vi "datatojson.vi"() -> (3 "json":string[](array[string]))   [LabVIEW 2016, in "工况数据上传.lvlib"]
panel:
  out "data":T1={"time"="2021-05-08 14-02-02", "data"={"ups"={"ups"={"input_voltage"=0.0, "input_frequency"=0.0, "output_voltage"=0.0, "output_current"=0.0, "output_frequency"=0.0, "output_active_power"=0.0, "output_apparent_power"=0.0, "load_rate"=0.0, "cabinet_temperature"=0.0, "battery_voltage"=0.0, "remaining_battery_capacity"=0.0, "power_on_status"="", "power_supply_mode"="", "fault"=FALSE, "battery_low_voltage"=FALSE, "mains_supply_abnormality"=FALSE}, "启用"=FALSE}, "air_conditioner"={"air_conditioner"={"cabinet_temperature"=0.0, "air_supply_temperature"=0.0, "voltage"=0.0, "current"=0.0, "compressor_status"="", "Internal_fan_status"="", "external_fan_status"="", "heating_state"="", "refrigeration_state"=FALSE, "high_temperature_alarm"=FALSE, "low_temperature_alarm"=FALSE, "heater_fault"=FALSE, "temperature_sensor_fault"=FALSE, "high_voltage_alarm"=FALSE, "low_voltage_alarm"=FALSE, "refrigeration_start_point"=0.0, "refrigeration_sensitive_point"=0.0, "heating_start_point"=0.0, "heating_sensitive_point"=0.0, "high_temperature_alarm_point"=0.0, "low_temperature_alarm_point"=0.0}, "启用"=FALSE}, "smoke_sensor"={"smoke_sensor"={"trigger_alarm"=FALSE}, "启用"=FALSE}, "water_immersion_sensor"={"water_immersion_sensor"={"trigger_alarm"=FALSE}, "启用"=FALSE}, "temperature_and_humidity_sensor"={"temperature_and_humidity_sensor"={"current_temperature"=0.0, "current_humidity"=0.0, "room_temperature_alarm"=FALSE, "humidity_alarm"=FALSE}, "启用"=FALSE}, "gps"={"gps"={"current_longitude"=0.0, "current_latitude"=0.0, "launch_longitude"=0.0, "launch_latitude"=0.0, "shift_alarm"=FALSE}, "启用"=FALSE}, "solar_controller"={"solar_controller"={"array_voltage"=0.0, "array_current"=0.0, "generating_power"=0.0, "battery_voltage"=0.0, "battery_current"=0.0, "ceiling_voltage"=0.0, "minimum_voltage"=0.0, "battery_temperature"=0.0, "remaining_battery_capacity"=0.0, "load_voltage"=0.0, "load_current"=0.0, "load_power"=0.0, "equipment_temperature"=0.0, "accumulated_electricity_consumption_of_the_day"=0.0, "accumulated_electricity_consumption_of_the_current_month"=0.0, "accumulated_electricity_consumption_in_the_current_year"=0.0, "total_accumulated_power_consumption"=0.0, "accumulated_charging_capacity_of_the_day"=0.0, "accumulated_charging_amount_of_the_current_month"=0.0, "accumulated_charging_capacity_of_the_current_year"=0.0, "total_cumulative_charge"=0.0}, "启用"=FALSE}, "solar_controller_2"={"solar_controller_2"={"array_voltage"=0.0, "array_current"=0.0, "generating_power"=0.0, "battery_voltage"=0.0, "battery_current"=0.0, "ceiling_voltage"=0.0, "minimum_voltage"=0.0, "battery_temperature"=0.0, "remaining_battery_capacity"=0.0, "load_voltage"=0.0, "load_current"=0.0, "load_power"=0.0, "equipment_temperature"=0.0, "accumulated_electricity_consumption_of_the_day"=0.0, "accumulated_electricity_consumption_of_the_current_month"=0.0, "accumulated_electricity_consumption_in_the_current_year"=0.0, "total_accumulated_power_consumption"=0.0, "accumulated_charging_capacity_of_the_day"=0.0, "accumulated_charging_amount_of_the_current_month"=0.0, "accumulated_charging_capacity_of_the_current_year"=0.0, "total_cumulative_charge"=0.0}, "启用"=FALSE}}} {"data"."air_conditioner"."air_conditioner"."current" format="%#.2g"}
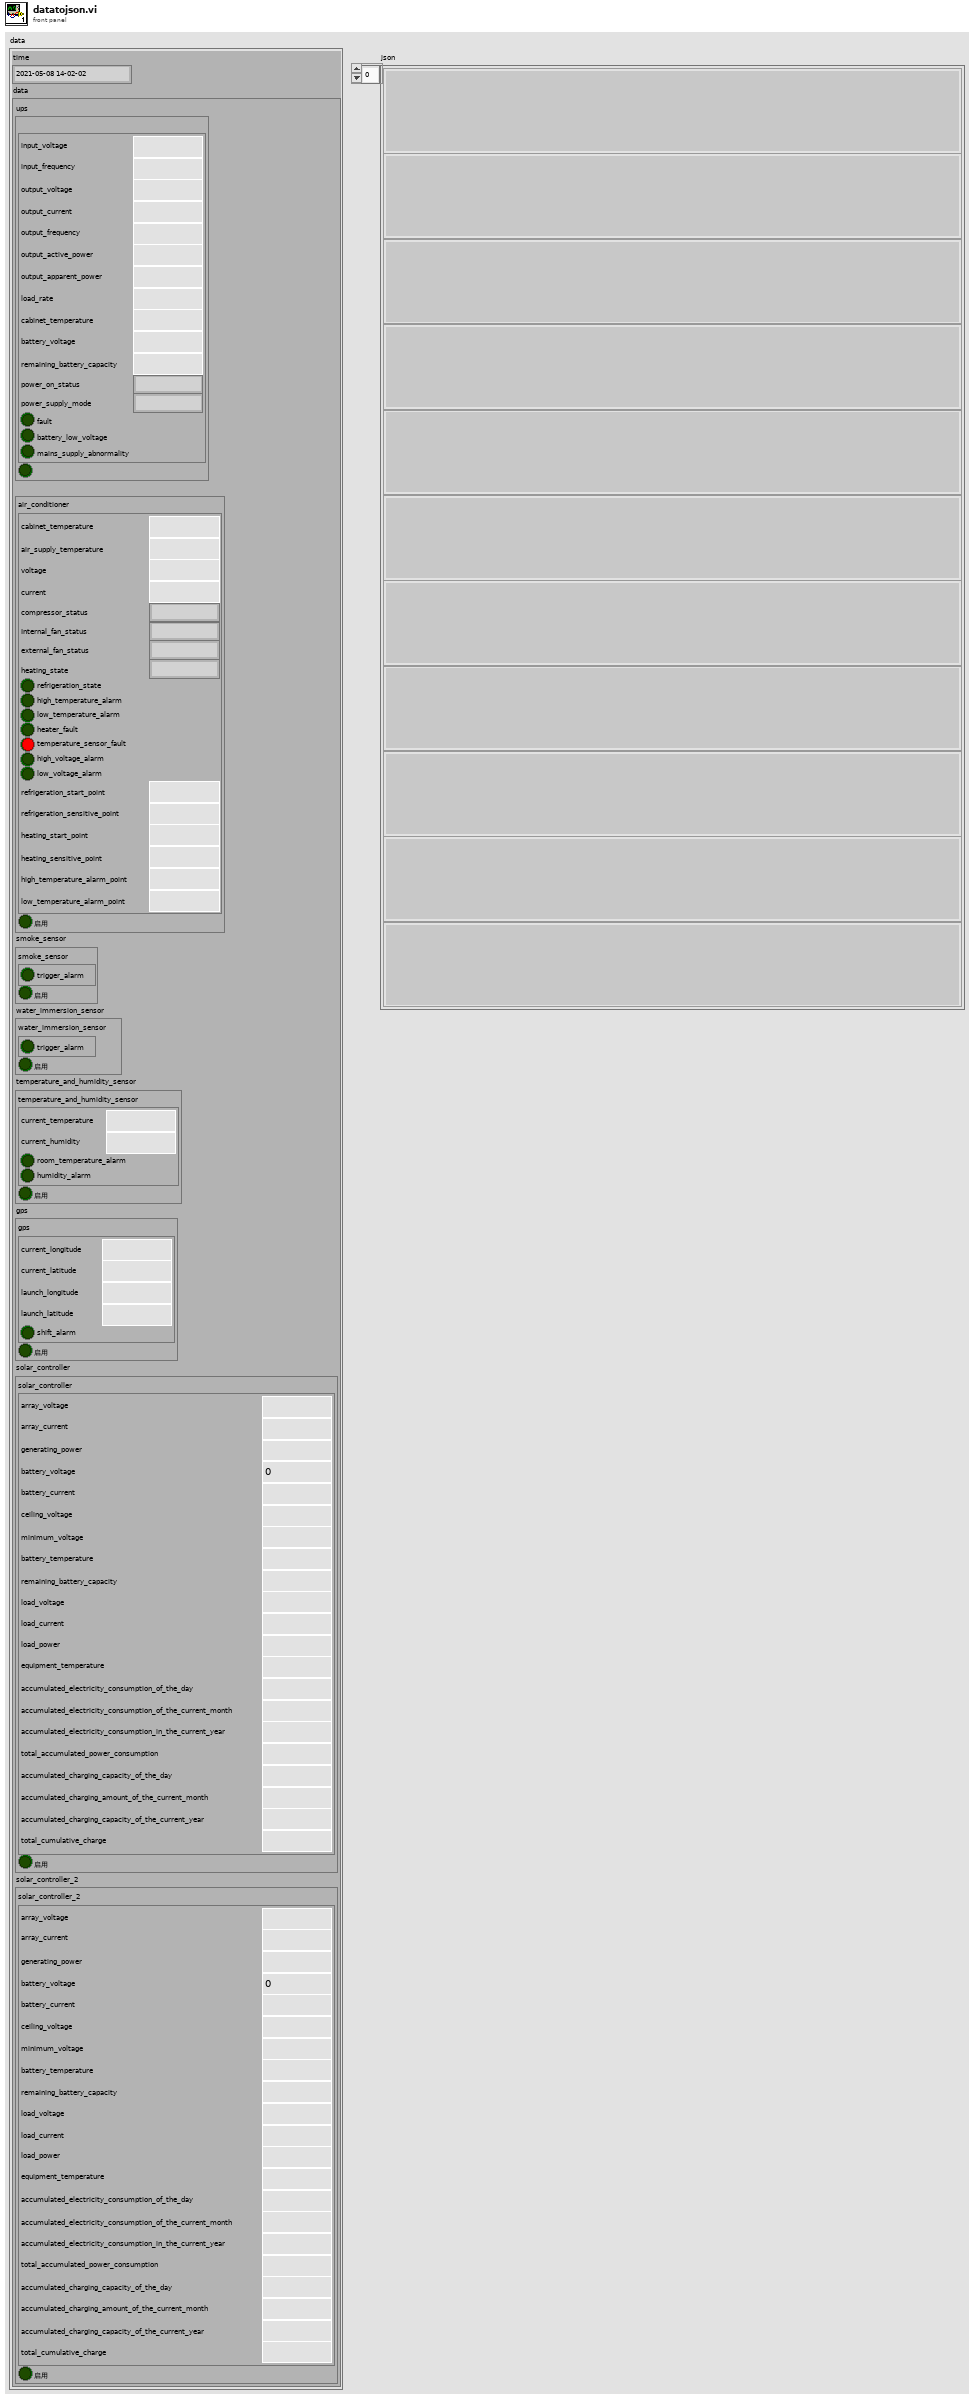
[diagram p1: front panel]
types:
  T1 = typedef "工况数据.ctl" = cluster{"time":string, "data":cluster{"ups":cluster{"ups":cluster{"input_voltage":ext, "input_frequency":ext, "output_voltage":ext, "output_current":ext, "output_frequency":ext, "output_active_power":ext, "output_apparent_power":ext, "load_rate":ext, "cabinet_temperature":ext, "battery_voltage":ext, "remaining_battery_capacity":ext, "power_on_status":string, "power_supply_mode":string, "fault":bool, "battery_low_voltage":bool, "mains_supply_abnormality":bool}, "启用":bool}, "air_conditioner":cluster{"air_conditioner":cluster{"cabinet_temperature":ext, "air_supply_temperature":ext, "voltage":ext, "current":ext, "compressor_status":string, "Internal_fan_status":string, "external_fan_status":string, "heating_state":string, "refrigeration_state":bool, "high_temperature_alarm":bool, "low_temperature_alarm":bool, "heater_fault":bool, "temperature_sensor_fault":bool, "high_voltage_alarm":bool, "low_voltage_alarm":bool, "refrigeration_start_point":ext, "refrigeration_sensitive_point":ext, "heating_start_point":ext, "heating_sensitive_point":ext, "high_temperature_alarm_point":ext, "low_temperature_alarm_point":ext}, "启用":bool}, "smoke_sensor":cluster{"smoke_sensor":cluster{"trigger_alarm":bool}, "启用":bool}, "water_immersion_sensor":cluster{"water_immersion_sensor":cluster{"trigger_alarm":bool}, "启用":bool}, "temperature_and_humidity_sensor":cluster{"temperature_and_humidity_sensor":cluster{"current_temperature":ext, "current_humidity":ext, "room_temperature_alarm":bool, "humidity_alarm":bool}, "启用":bool}, "gps":cluster{"gps":cluster{"current_longitude":ext, "current_latitude":ext, "launch_longitude":ext, "launch_latitude":ext, "shift_alarm":bool}, "启用":bool}, "solar_controller":cluster{"solar_controller":cluster{"array_voltage":ext, "array_current":ext, "generating_power":ext, "battery_voltage":dbl, "battery_current":ext, "ceiling_voltage":ext, "minimum_voltage":ext, "battery_temperature":ext, "remaining_battery_capacity":ext, "load_voltage":ext, "load_current":ext, "load_power":ext, "equipment_temperature":ext, "accumulated_electricity_consumption_of_the_day":ext, "accumulated_electricity_consumption_of_the_current_month":ext, "accumulated_electricity_consumption_in_the_current_year":ext, "total_accumulated_power_consumption":ext, "accumulated_charging_capacity_of_the_day":ext, "accumulated_charging_amount_of_the_current_month":ext, "accumulated_charging_capacity_of_the_current_year":ext, "total_cumulative_charge":ext}, "启用":bool}, "solar_controller_2":cluster{"solar_controller_2":cluster{"array_voltage":ext, "array_current":ext, "generating_power":ext, "battery_voltage":dbl, "battery_current":ext, "ceiling_voltage":ext, "minimum_voltage":ext, "battery_temperature":ext, "remaining_battery_capacity":ext, "load_voltage":ext, "load_current":ext, "load_power":ext, "equipment_temperature":ext, "accumulated_electricity_consumption_of_the_day":ext, "accumulated_electricity_consumption_of_the_current_month":ext, "accumulated_electricity_consumption_in_the_current_year":ext, "total_accumulated_power_consumption":ext, "accumulated_charging_capacity_of_the_day":ext, "accumulated_charging_amount_of_the_current_month":ext, "accumulated_charging_capacity_of_the_current_year":ext, "total_cumulative_charge":ext}, "启用":bool}}}
  T2 = cluster{"ups":cluster{"ups":cluster{"input_voltage":ext, "input_frequency":ext, "output_voltage":ext, "output_current":ext, "output_frequency":ext, "output_active_power":ext, "output_apparent_power":ext, "load_rate":ext, "cabinet_temperature":ext, "battery_voltage":ext, "remaining_battery_capacity":ext, "power_on_status":string, "power_supply_mode":string, "fault":bool, "battery_low_voltage":bool, "mains_supply_abnormality":bool}, "启用":bool}, "air_conditioner":cluster{"air_conditioner":cluster{"cabinet_temperature":ext, "air_supply_temperature":ext, "voltage":ext, "current":ext, "compressor_status":string, "Internal_fan_status":string, "external_fan_status":string, "heating_state":string, "refrigeration_state":bool, "high_temperature_alarm":bool, "low_temperature_alarm":bool, "heater_fault":bool, "temperature_sensor_fault":bool, "high_voltage_alarm":bool, "low_voltage_alarm":bool, "refrigeration_start_point":ext, "refrigeration_sensitive_point":ext, "heating_start_point":ext, "heating_sensitive_point":ext, "high_temperature_alarm_point":ext, "low_temperature_alarm_point":ext}, "启用":bool}, "smoke_sensor":cluster{"smoke_sensor":cluster{"trigger_alarm":bool}, "启用":bool}, "water_immersion_sensor":cluster{"water_immersion_sensor":cluster{"trigger_alarm":bool}, "启用":bool}, "temperature_and_humidity_sensor":cluster{"temperature_and_humidity_sensor":cluster{"current_temperature":ext, "current_humidity":ext, "room_temperature_alarm":bool, "humidity_alarm":bool}, "启用":bool}, "gps":cluster{"gps":cluster{"current_longitude":ext, "current_latitude":ext, "launch_longitude":ext, "launch_latitude":ext, "shift_alarm":bool}, "启用":bool}, "solar_controller":cluster{"solar_controller":cluster{"array_voltage":ext, "array_current":ext, "generating_power":ext, "battery_voltage":dbl, "battery_current":ext, "ceiling_voltage":ext, "minimum_voltage":ext, "battery_temperature":ext, "remaining_battery_capacity":ext, "load_voltage":ext, "load_current":ext, "load_power":ext, "equipment_temperature":ext, "accumulated_electricity_consumption_of_the_day":ext, "accumulated_electricity_consumption_of_the_current_month":ext, "accumulated_electricity_consumption_in_the_current_year":ext, "total_accumulated_power_consumption":ext, "accumulated_charging_capacity_of_the_day":ext, "accumulated_charging_amount_of_the_current_month":ext, "accumulated_charging_capacity_of_the_current_year":ext, "total_cumulative_charge":ext}, "启用":bool}, "solar_controller_2":cluster{"solar_controller_2":cluster{"array_voltage":ext, "array_current":ext, "generating_power":ext, "battery_voltage":dbl, "battery_current":ext, "ceiling_voltage":ext, "minimum_voltage":ext, "battery_temperature":ext, "remaining_battery_capacity":ext, "load_voltage":ext, "load_current":ext, "load_power":ext, "equipment_temperature":ext, "accumulated_electricity_consumption_of_the_day":ext, "accumulated_electricity_consumption_of_the_current_month":ext, "accumulated_electricity_consumption_in_the_current_year":ext, "total_accumulated_power_consumption":ext, "accumulated_charging_capacity_of_the_day":ext, "accumulated_charging_amount_of_the_current_month":ext, "accumulated_charging_capacity_of_the_current_year":ext, "total_cumulative_charge":ext}, "启用":bool}}
  T3 = cluster{"ups":cluster{"input_voltage":ext, "input_frequency":ext, "output_voltage":ext, "output_current":ext, "output_frequency":ext, "output_active_power":ext, "output_apparent_power":ext, "load_rate":ext, "cabinet_temperature":ext, "battery_voltage":ext, "remaining_battery_capacity":ext, "power_on_status":string, "power_supply_mode":string, "fault":bool, "battery_low_voltage":bool, "mains_supply_abnormality":bool}, "启用":bool}
  T4 = cluster{"air_conditioner":cluster{"cabinet_temperature":ext, "air_supply_temperature":ext, "voltage":ext, "current":ext, "compressor_status":string, "Internal_fan_status":string, "external_fan_status":string, "heating_state":string, "refrigeration_state":bool, "high_temperature_alarm":bool, "low_temperature_alarm":bool, "heater_fault":bool, "temperature_sensor_fault":bool, "high_voltage_alarm":bool, "low_voltage_alarm":bool, "refrigeration_start_point":ext, "refrigeration_sensitive_point":ext, "heating_start_point":ext, "heating_sensitive_point":ext, "high_temperature_alarm_point":ext, "low_temperature_alarm_point":ext}, "启用":bool}
  T5 = cluster{"smoke_sensor":cluster{"trigger_alarm":bool}, "启用":bool}
  T6 = cluster{"water_immersion_sensor":cluster{"trigger_alarm":bool}, "启用":bool}
  T7 = cluster{"temperature_and_humidity_sensor":cluster{"current_temperature":ext, "current_humidity":ext, "room_temperature_alarm":bool, "humidity_alarm":bool}, "启用":bool}
  T8 = cluster{"gps":cluster{"current_longitude":ext, "current_latitude":ext, "launch_longitude":ext, "launch_latitude":ext, "shift_alarm":bool}, "启用":bool}
  T9 = cluster{"solar_controller":cluster{"array_voltage":ext, "array_current":ext, "generating_power":ext, "battery_voltage":dbl, "battery_current":ext, "ceiling_voltage":ext, "minimum_voltage":ext, "battery_temperature":ext, "remaining_battery_capacity":ext, "load_voltage":ext, "load_current":ext, "load_power":ext, "equipment_temperature":ext, "accumulated_electricity_consumption_of_the_day":ext, "accumulated_electricity_consumption_of_the_current_month":ext, "accumulated_electricity_consumption_in_the_current_year":ext, "total_accumulated_power_consumption":ext, "accumulated_charging_capacity_of_the_day":ext, "accumulated_charging_amount_of_the_current_month":ext, "accumulated_charging_capacity_of_the_current_year":ext, "total_cumulative_charge":ext}, "启用":bool}
  T10 = cluster{"solar_controller_2":cluster{"array_voltage":ext, "array_current":ext, "generating_power":ext, "battery_voltage":dbl, "battery_current":ext, "ceiling_voltage":ext, "minimum_voltage":ext, "battery_temperature":ext, "remaining_battery_capacity":ext, "load_voltage":ext, "load_current":ext, "load_power":ext, "equipment_temperature":ext, "accumulated_electricity_consumption_of_the_day":ext, "accumulated_electricity_consumption_of_the_current_month":ext, "accumulated_electricity_consumption_in_the_current_year":ext, "total_accumulated_power_consumption":ext, "accumulated_charging_capacity_of_the_day":ext, "accumulated_charging_amount_of_the_current_month":ext, "accumulated_charging_capacity_of_the_current_year":ext, "total_cumulative_charge":ext}, "启用":bool}
  T11 = cluster{"current_temperature":ext, "current_humidity":ext, "room_temperature_alarm":bool, "humidity_alarm":bool}
  T12 = cluster{"array_voltage":ext, "array_current":ext, "generating_power":ext, "battery_voltage":dbl, "battery_current":ext, "ceiling_voltage":ext, "minimum_voltage":ext, "battery_temperature":ext, "remaining_battery_capacity":ext, "load_voltage":ext, "load_current":ext, "load_power":ext, "equipment_temperature":ext, "accumulated_electricity_consumption_of_the_day":ext, "accumulated_electricity_consumption_of_the_current_month":ext, "accumulated_electricity_consumption_in_the_current_year":ext, "total_accumulated_power_consumption":ext, "accumulated_charging_capacity_of_the_day":ext, "accumulated_charging_amount_of_the_current_month":ext, "accumulated_charging_capacity_of_the_current_year":ext, "total_cumulative_charge":ext}
  T13 = cluster{"cabinet_temperature":ext, "air_supply_temperature":ext, "voltage":ext, "current":ext, "compressor_status":string, "Internal_fan_status":string, "external_fan_status":string, "heating_state":string, "refrigeration_state":bool, "high_temperature_alarm":bool, "low_temperature_alarm":bool, "heater_fault":bool, "temperature_sensor_fault":bool, "high_voltage_alarm":bool, "low_voltage_alarm":bool, "refrigeration_start_point":ext, "refrigeration_sensitive_point":ext, "heating_start_point":ext, "heating_sensitive_point":ext, "high_temperature_alarm_point":ext, "low_temperature_alarm_point":ext}
  T14 = cluster{"input_voltage":ext, "input_frequency":ext, "output_voltage":ext, "output_current":ext, "output_frequency":ext, "output_active_power":ext, "output_apparent_power":ext, "load_rate":ext, "cabinet_temperature":ext, "battery_voltage":ext, "remaining_battery_capacity":ext, "power_on_status":string, "power_supply_mode":string, "fault":bool, "battery_low_voltage":bool, "mains_supply_abnormality":bool}
  T15 = cluster{"current_longitude":ext, "current_latitude":ext, "launch_longitude":ext, "launch_latitude":ext, "shift_alarm":bool}
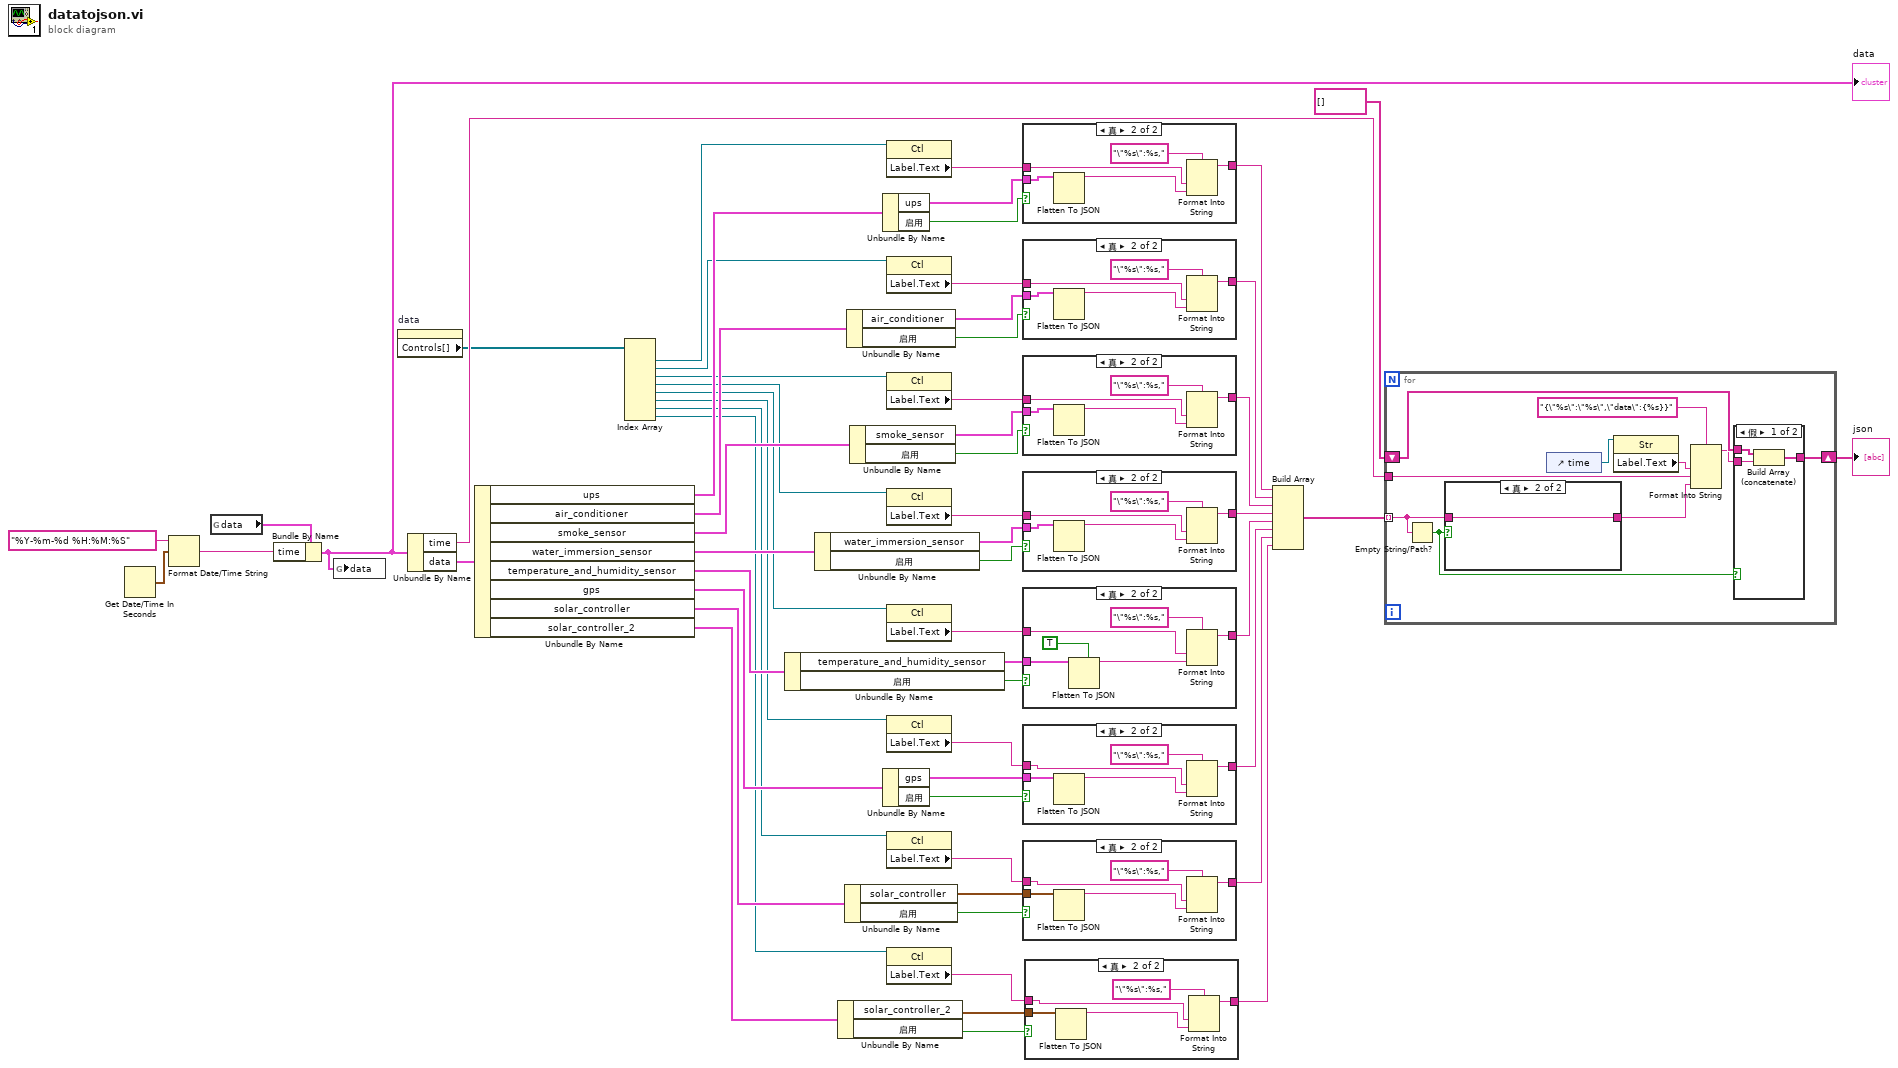
[diagram p0: block diagram]
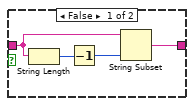
[diagram p3: hidden frame]
diagram:
  n1 = Get Date/Time In Seconds() -> (seconds since 1Jan1904=w18:timestamp)
  n2 = Format Date/Time String(time format string (%c)="%Y-%m-%d %H:%M:%S" ("时间格式字符串(%c)"), seconds (now)=w18) -> (date/time string=w16:string)  [unwired: 1 in]
  n3 = global read "工况数据接口全局.vi" "data"() -> (w17:T1)
  n4 = Bundle By Name(cluster=w17, "time"=w16) -> (w12:T1)
  "data" <- w12
  n5 = global write "工况数据接口全局.vi" "data"(w12) -> ()
  n6 = property on="data" class="Clust (严格)"() -> ("Controls[]"=w13:refnum<vi>[])  [unwired: 2 in, 2 out]
  n7 = Unbundle By Name(w12) -> ("time"=w15:string, "data"=w14:T2)
  n8 = Unbundle By Name(w14) -> ("ups"=w59:T3, "air_conditioner"=w54:T4, "smoke_sensor"=w45:T5, "water_immersion_sensor"=w40:T6, "temperature_and_humidity_sensor"=w36:T7, "gps"=w31:T8, "solar_controller"=w25:T9, "solar_controller_2"=w20:T10)
  n9 = Index Array(array=w13) -> (element #1=w57:refnum<vi>, element #2=w51:refnum<vi>, element #3=w46:refnum<vi>, element #4=w41:refnum<vi>, element #5=w35:refnum<vi>, element #6=w30:refnum<vi>, element #7=w26:refnum<vi>, element #8=w21:refnum<vi>)  [unwired: 8 in]
  n10 = Unbundle By Name(w36) -> ("temperature_and_humidity_sensor"=w38:T11, "启用"=w39:bool)
  n11 = Unbundle By Name(w40) -> ("water_immersion_sensor"=w43:cluster{"trigger_alarm":bool}, "启用"=w44:bool)
  n12 = Unbundle By Name(w20) -> ("solar_controller_2"=w23:T12, "启用"=w24:bool)
  n13 = Unbundle By Name(w25) -> ("solar_controller"=w28:T12, "启用"=w29:bool)
  n14 = Unbundle By Name(w54) -> ("air_conditioner"=w52:T13, "启用"=w53:bool)
  n15 = Unbundle By Name(w45) -> ("smoke_sensor"=w48:cluster{"trigger_alarm":bool}, "启用"=w47:bool)
  n16 = Unbundle By Name(w59) -> ("ups"=w58:T14, "启用"=w55:bool)
  n17 = Unbundle By Name(w31) -> ("gps"=w33:T15, "启用"=w34:bool)
  n18 = property class="Ctl"(reference=w57) -> ("Label.Text"=w56:string)  [unwired: 1 in, 2 out]
  n19 = property class="Ctl"(reference=w51) -> ("Label.Text"=w50:string)  [unwired: 1 in, 2 out]
  n20 = property class="Ctl"(reference=w46) -> ("Label.Text"=w49:string)  [unwired: 1 in, 2 out]
  n21 = property class="Ctl"(reference=w41) -> ("Label.Text"=w42:string)  [unwired: 1 in, 2 out]
  n22 = property class="Ctl"(reference=w35) -> ("Label.Text"=w37:string)  [unwired: 1 in, 2 out]
  n23 = property class="Ctl"(reference=w30) -> ("Label.Text"=w32:string)  [unwired: 1 in, 2 out]
  n24 = property class="Ctl"(reference=w26) -> ("Label.Text"=w27:string)  [unwired: 1 in, 2 out]
  n25 = property class="Ctl"(reference=w21) -> ("Label.Text"=w22:string)  [unwired: 1 in, 2 out]
  n26 = case shown="真" w55 {
    tunnel: w58 -> [_ w64]
    tunnel: w56 -> [_ w62]
    tunnel: [_ w61] -> w11
    frame False {
    }
    frame True {
      n27 = Flatten To JSON(anything=w64) -> (JSON string=w60:string)  [unwired: 2 in, 1 out]
      n28 = Format Into String(format string="\"%s\":%s," ("格式字符串"), w62, w60) -> (resulting string=w61:string)  [unwired: 2 in, 1 out]
    }
  }
  n29 = case shown="真" w53 {
    tunnel: w52 -> [_ w69]
    tunnel: w50 -> [_ w67]
    tunnel: [_ w66] -> w10
    frame False {
    }
    frame True {
      n30 = Flatten To JSON(anything=w69) -> (JSON string=w65:string)  [unwired: 2 in, 1 out]
      n31 = Format Into String(format string="\"%s\":%s," ("格式字符串"), w67, w65) -> (resulting string=w66:string)  [unwired: 2 in, 1 out]
    }
  }
  n32 = case shown="真" w47 {
    tunnel: w48 -> [_ w74]
    tunnel: w49 -> [_ w72]
    tunnel: [_ w71] -> w9
    frame False {
    }
    frame True {
      n33 = Flatten To JSON(anything=w74) -> (JSON string=w70:string)  [unwired: 2 in, 1 out]
      n34 = Format Into String(format string="\"%s\":%s," ("格式字符串"), w72, w70) -> (resulting string=w71:string)  [unwired: 2 in, 1 out]
    }
  }
  n35 = case shown="真" w44 {
    tunnel: w43 -> [_ w79]
    tunnel: w42 -> [_ w77]
    tunnel: [_ w76] -> w8
    frame False {
    }
    frame True {
      n36 = Flatten To JSON(anything=w79) -> (JSON string=w75:string)  [unwired: 2 in, 1 out]
      n37 = Format Into String(format string="\"%s\":%s," ("格式字符串"), w77, w75) -> (resulting string=w76:string)  [unwired: 2 in, 1 out]
    }
  }
  n38 = case shown="真" w39 {
    tunnel: w38 -> [_ w85]
    tunnel: w37 -> [_ w83]
    tunnel: [_ w82] -> w7
    frame False {
    }
    frame True {
      n39 = Flatten To JSON(enable LabVIEW extensions? (T)=TRUE ("启用LabVIEW扩展？(T)"), anything=w85) -> (JSON string=w81:string)  [unwired: 1 in, 1 out]
      n40 = Format Into String(format string="\"%s\":%s," ("格式字符串"), w83, w81) -> (resulting string=w82:string)  [unwired: 2 in, 1 out]
    }
  }
  n41 = case shown="真" w34 {
    tunnel: w33 -> [_ w90]
    tunnel: w32 -> [_ w88]
    tunnel: [_ w87] -> w6
    frame False {
    }
    frame True {
      n42 = Flatten To JSON(anything=w90) -> (JSON string=w86:string)  [unwired: 2 in, 1 out]
      n43 = Format Into String(format string="\"%s\":%s," ("格式字符串"), w88, w86) -> (resulting string=w87:string)  [unwired: 2 in, 1 out]
    }
  }
  n44 = case shown="真" w29 {
    tunnel: w28 -> [_ w95]
    tunnel: w27 -> [_ w93]
    tunnel: [_ w92] -> w5
    frame False {
    }
    frame True {
      n45 = Flatten To JSON(anything=w95) -> (JSON string=w91:string)  [unwired: 2 in, 1 out]
      n46 = Format Into String(format string="\"%s\":%s," ("格式字符串"), w93, w91) -> (resulting string=w92:string)  [unwired: 2 in, 1 out]
    }
  }
  n47 = case shown="真" w24 {
    tunnel: w23 -> [_ w100]
    tunnel: w22 -> [_ w98]
    tunnel: [_ w97] -> w4
    frame False {
    }
    frame True {
      n48 = Flatten To JSON(anything=w100) -> (JSON string=w96:string)  [unwired: 2 in, 1 out]
      n49 = Format Into String(format string="\"%s\":%s," ("格式字符串"), w98, w96) -> (resulting string=w97:string)  [unwired: 2 in, 1 out]
    }
  }
  n50 = Build Array(w11, w10, w9, w8, w7, w6, w5, w4) -> (w3:string[])
  n51 = for {
    tunnel: w15 -> [w108]
    tunnel: w3 -> [w105] mode=indexing
    shift-right: [w102] -> w1
    shift-left: string[] [] ("json") -> [w104]
    n52 = Empty String/Path?(string/path=w105) -> (empty?=w101:bool)
    n53 = case shown="真" w101 {
      tunnel: w105 -> [w118 w119]
      tunnel: [w115 w119] -> w106
      frame False {
        n54 = String Length(string=w118) -> (length=w117:i32)
        n55 = Decrement(x=w117) -> (x-1=w116:i32)
        n56 = String Subset(string=w118, length (rest)=w116) -> (substring=w115:string)  [unwired: 1 in]
      }
      frame True {
      }
    }
    n57 = control-ref of="time"() -> (w107:refnum<vi>)
    n58 = property class="Str"(reference=w107) -> ("Label.Text"=w109:string)  [unwired: 1 in, 2 out]
    n59 = Format Into String(format string="{\"%s\":\"%s\",\"data\":{%s}}" ("格式字符串"), w109, w108, w106) -> (resulting string=w103:string)  [unwired: 2 in, 1 out]
    n60 = case shown="假" w101 {
      tunnel: w104 -> [w113 w114]
      tunnel: w103 -> [w112 _]
      tunnel: [w111 w114] -> w102
      frame False {
        n61 = Build Array (concatenate)(w113, w112) -> (w111:string[])
      }
      frame True {
      }
    }
  }
  "json" <- w1
